vi "Legendbox in pie.vi"(9 "Width":u32, 10 "Last Text":T1, 11 "Gap":i32) -> (2 "New Text":T1)   [LabVIEW 2019, in "Zen Analytics.lvlib" / "Zen Analytics.lvclass"]
uses:
  Zen Analytics.lvclass
types:
  T1 = cluster{"left":i16, "top":i16, "right":i16, "bottom":i16}
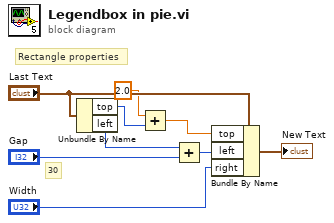
[diagram p0: block diagram]
diagram:
  # "30"
  # "Rectangle properties"
  n1 = Unbundle By Name("Last Text") -> ("top"=w8:i16, "left"=w4:i16)
  n2 = Add(x=2.0 ("y"), y=w8) -> (x+y=w9:dbl)
  n3 = Add(x=w4, y="Gap") -> (x+y=w5:i32)
  n4 = Bundle By Name(cluster="Last Text", "top"=w9, "left"=w5, "right"="Width") -> (→"New Text":T1)
